vi "ScriptEngineMutex.vi"(9 "Priority":u8, 10 "Calling Script":string, 11 "Mutex Mode":T2=enum."Request Execution") -> (3 "Mutex State":T1)   [LabVIEW 2011]
uses:
  MutexMode.ctl
  MutexState.ctl
panel:
  # "Script Engine Mutex manages the locking and usage of the script engine, since it is not multi-threaded."
  # "It also asynchronously launches the script engine when a non-auto script is requested"
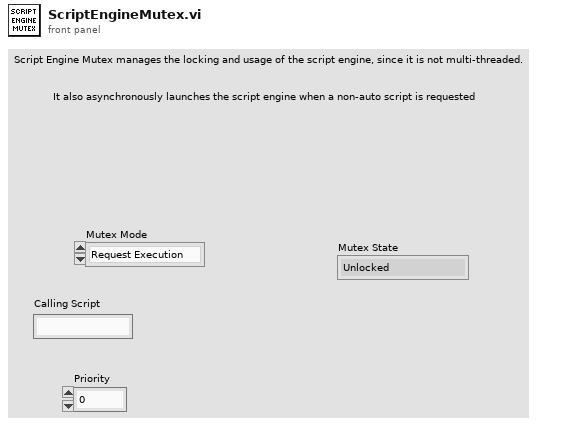
[diagram p1: front panel]
types:
  T1 = typedef "MutexState.ctl" = enum16{"Unlocked", "Locked-You", "Locked-Unknown", "Locked-ScriptButton", "Locked-Autonomous"}
  T2 = typedef "MutexMode.ctl" = enum16{"Get Mode", "Request Execution", "Stop Execution", "Lock Autonomous", "Script Completed"}
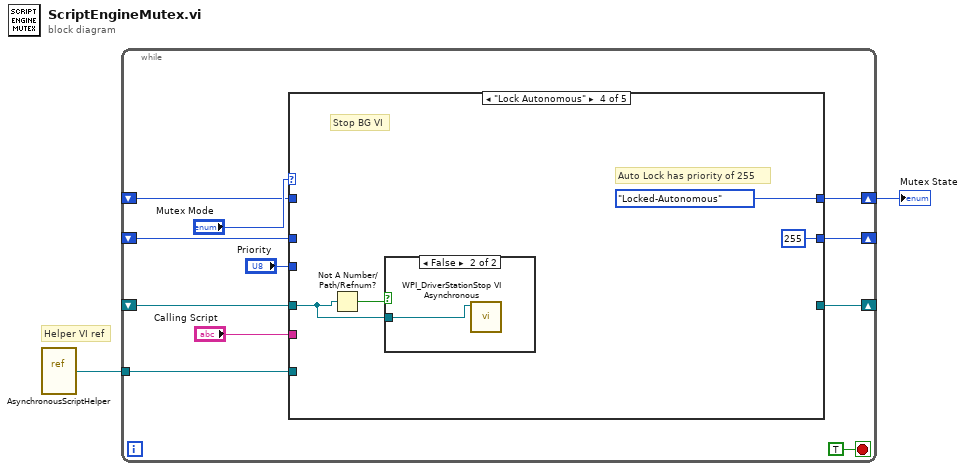
[diagram p0: block diagram]
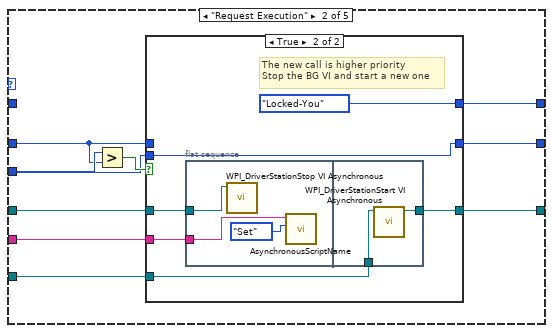
[diagram p3: hidden frame]
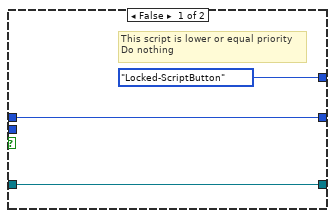
[diagram p4: hidden frame]
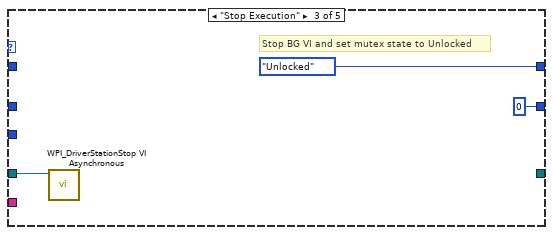
[diagram p5: hidden frame]
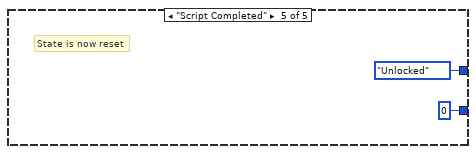
[diagram p7: hidden frame]
diagram:
  # "Helper VI ref"
  n1 = vi-ref "AsynchronousScriptHelper.vi"() -> (w1:refnum<vi>)
  n2 = while {
    shift-right: [w11] -> w2
    shift-left: _ -> [w10]
    shift-right: [w3] -> _
    shift-left: _ -> [w8]
    shift-right: [w4] -> _
    shift-left: _ -> [w7]
    tunnel: w1 -> [w5]
    stop <- TRUE stop-if-true
    n3 = case shown="\"Lock Autonomous\"" "Mutex Mode" {
      tunnel: [w16 w20 MutexState."Unlocked" ("Mutex State") MutexState."Locked-Autonomous" ("Mutex State") MutexState."Unlocked" ("Mutex State")] -> w11
      tunnel: w10 -> [w16 _ _ _ _]
      tunnel: "Priority" -> [_ w18 _ _ _]
      tunnel: w8 -> [w15 w17 _ _ _]
      tunnel: w7 -> [w14 w24 w40 w43 _]
      tunnel: "Calling Script" -> [_ w23 _ _ _]
      tunnel: w5 -> [_ w22 _ _ _]
      tunnel: [w14 w21 _ _ _] -> w4
      tunnel: [w15 w19 u8 0 ("Priority") u8 255 ("Priority") u8 0 ("Priority")] -> w3
      frame "Get Mode", Default {
        # "Do nothing, they'll read it as they want"
      }
      frame "Request Execution" {
        n4 = Greater?(x=w18, y=w17) -> (0:w25:bool)
        n5 = case shown="True" w25 {
          tunnel: w24 -> [w28 w34]
          tunnel: w23 -> [_ w33]
          tunnel: w22 -> [_ w32]
          tunnel: [w28 w31] -> w21
          tunnel: [MutexState."Locked-ScriptButton" ("Mutex State") MutexState."Locked-You" ("Mutex State")] -> w20
          tunnel: [w27 w29] -> w19
          tunnel: w17 -> [w27 _]
          tunnel: w18 -> [_ w29]
          frame False {
            # "This script is lower or equal priority\nDo nothing"
          }
          frame True {
            # "The new call is higher priority\nStop the BG VI and start a new one"
            n6 = flat-sequence {
              tunnel: w34 -> [w37]
              tunnel: w33 -> [w35]
              tunnel: w32 -> [w39]
              tunnel: [w38] -> w31
              frame #0 {
                n7 = call <vilib>:"WPI_DriverStationStop VI Asynchronous.vi"("VI Refnum"=w37) -> ()  [unwired: 11 out]
                n8 = call "AsynchronousScriptName.vi"("data_store_mode"=enum16{"Set", "Get"}."Set", "Call Script"=w35) -> ()  [unwired: 9 in, 1 out]
              }
              frame #1 {
                n9 = call <vilib>:"WPI_DriverStationStart VI Asynchronous.vi"("VI"=w39) -> ("VI out"=w38:refnum<vi>)  [unwired: 10 out]
              }
            }
          }
        }
      }
      frame "Stop Execution" {
        # "Stop BG VI and set mutex state to Unlocked"
        n10 = call <vilib>:"WPI_DriverStationStop VI Asynchronous.vi"("VI Refnum"=w40) -> ()  [unwired: 11 out]
      }
      frame "Lock Autonomous" {
        # "Stop BG VI"
        # "Auto Lock has priority of 255"
        n11 = Not A Number/Path/Refnum?(number/path/refnum=w43) -> (NaN/Path/Refnum?=w44:bool)
        n12 = case shown="False" w44 {
          tunnel: w43 -> [_ w47]
          frame True {
          }
          frame False {
            n13 = call <vilib>:"WPI_DriverStationStop VI Asynchronous.vi"("VI Refnum"=w47) -> ()  [unwired: 11 out]
          }
        }
      }
      frame "Script Completed" {
        # "State is now reset"
      }
    }
  }
  "Mutex State" <- w2
